vi "CANOpen_Format dynamicSDO to String Array.vi"(7 "Display format":T1=enum."Decimal", 8 "error in (no error)":errorcluster, 11 "SDO Parameters":T2[](array[typedef]) {"Sub-Index (0)" format="%.0x"; "Object Index" format="%.0x"; "Block Data" format="%.0x"}) -> (0 "error out":errorcluster, 3 "Array":string[][](array[string]))   [LabVIEW 2021, in "CANOpen Addon System Explorer.lvlib"]
uses:
  CANOpen Addon System Explorer.lvlib
  Shared/CANOpen_SDO Settings.ctl
  CANOpen_SDO data format.ctl
  Shared/CANOpen Addon Shared.lvlib
panel:
  # "LSB"
  # "MSB"
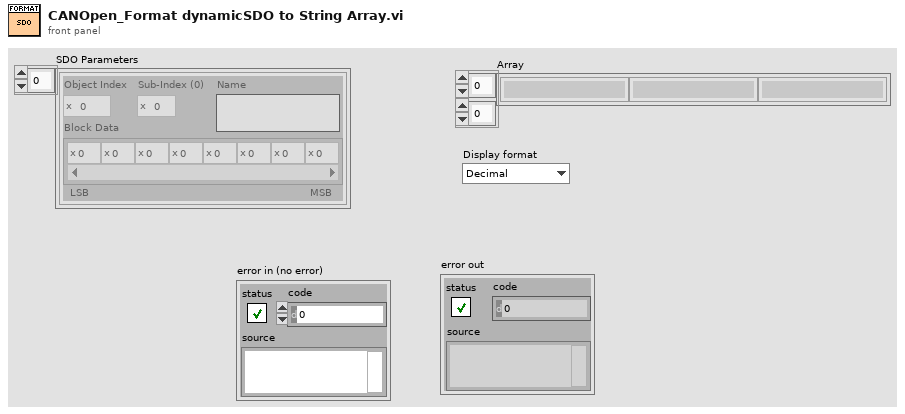
[diagram p1: front panel]
types:
  T1 = typedef "CANOpen Addon System Explorer.lvlib/CANOpen_SDO data format.ctl" = enum16{"Hexadecimal", "Decimal"}
  T2 = typedef "CANOpen Addon Shared.lvlib/CANOpen_SDO Settings.ctl" = cluster{"Object Index":u16, "Sub-Index (0)":u8, "Block Data":u8[], "Name":string}
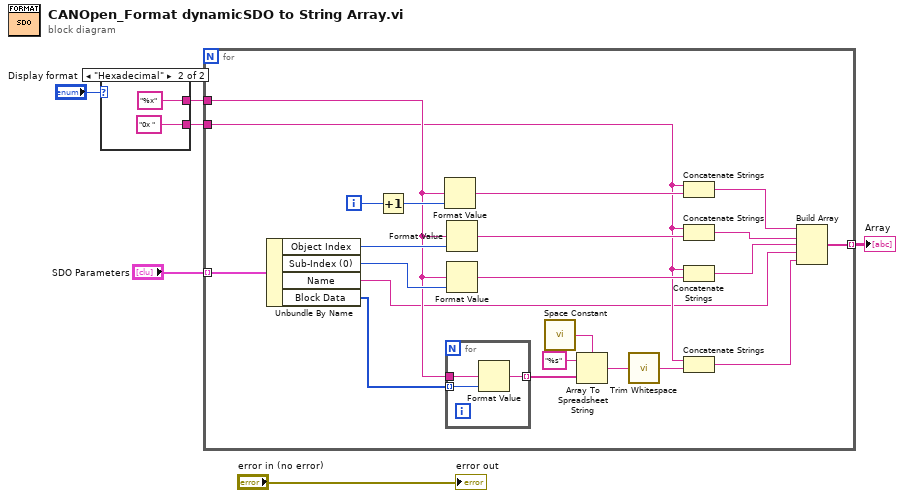
[diagram p0: block diagram]
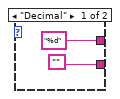
[diagram p2: hidden frame]
diagram:
  n1 = case shown="\"Hexadecimal\"" "Display format" {
    tunnel: ["%d" "%x"] -> w5
    tunnel: ["" "0x "] -> w1
    frame "Decimal" {
    }
    frame "Hexadecimal" {
    }
  }
  n2 = for {
    tunnel: "SDO Parameters" -> [w32] mode=indexing
    tunnel: w5 -> [w22]
    tunnel: [w25] -> w3 mode=indexing
    tunnel: w1 -> [w17]
    i -> [w24]
    n3 = Unbundle By Name(w32) -> ("Object Index"=w30:u16, "Sub-Index (0)"=w31:u8, "Name"=w12:string, "Block Data"=w11:u8[])
    n4 = Increment(x=w24) -> (x+1=w23:i32)
    n5 = Format Value(format string=w22, value (0)=w23) -> (output string=w18:string)  [unwired: 1 in]
    n6 = for {
      tunnel: w11 -> [w35] mode=indexing
      tunnel: w22 -> [w34]
      tunnel: [w33] -> w29 mode=indexing
      n7 = Format Value(format string=w34, value (0)=w35) -> (output string=w33:string)  [unwired: 1 in]
    }
    n8 = Format Value(format string=w22, value (0)=w30) -> (output string=w19:string)  [unwired: 1 in]
    n9 = Format Value(format string=w22, value (0)=w31) -> (output string=w20:string)  [unwired: 1 in]
    n10 = call <vilib>:"Space Constant.vi"() -> ("String"=w27:string)
    n11 = Array To Spreadsheet String(delimiter (Tab)=w27, array=w29, 3:"%s" ("format string")) -> (spreadsheet string=w26:string)
    n12 = call <vilib>:"Trim Whitespace.vi"("string"=w26) -> ("trimmed string"=w21:string)  [unwired: 1 in]
    n13 = Concatenate Strings(w17, w18) -> (w16:string)
    n14 = Concatenate Strings(w17, w19) -> (w15:string)
    n15 = Concatenate Strings(w17, w20) -> (w14:string)
    n16 = Concatenate Strings(w17, w21) -> (w13:string)
    n17 = Build Array(w16, w15, w14, w12, w13) -> (w25:string[])
  }
  "Array" <- w3
  "error out" <- "error in (no error)"
